vi "Planta de Nivel.vi"() -> ()   [LabVIEW 2020]
uses:
  <vilib>/NI/Modbus Library/API/Wrapper/Create TCP Master.vi
  <vilib>/ErrorRing/Error Ring.xnode
  <vilib>/NI/Modbus Library/API/Master/Modbus Master.lvclass
  <vilib>/NI/Modbus Library/API/Wrapper/API Main.lvlib
panel:
  in  "Vertical Progress Bar":u16(slide) scale=0.0..10.0
  in  "stop":bool
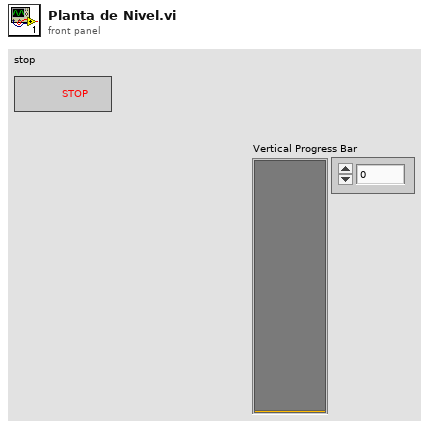
[diagram p1: front panel]
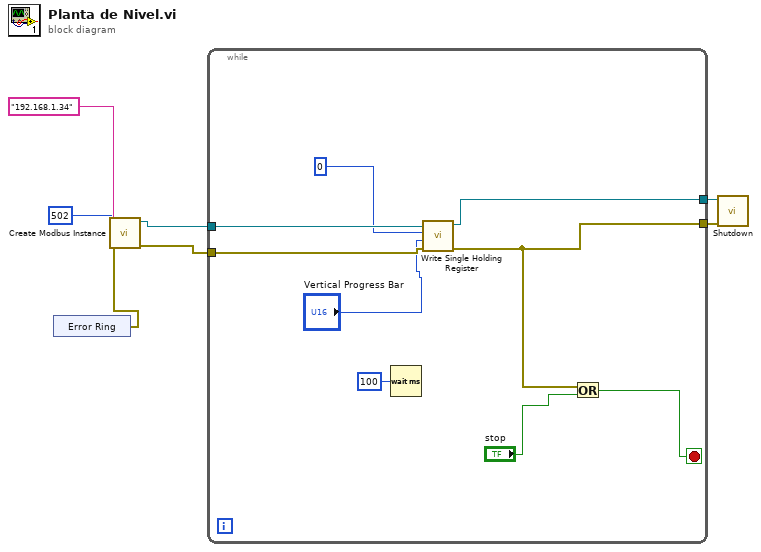
[diagram p0: block diagram]
diagram:
  n1 = xnode "Error Ring"() -> ("error out"=w1:errorcluster)
  n2 = call-poly <vilib>:"Create Modbus Instance.vi"("error in"=w1, "port (502)"=u16 502, "address"="192.168.1.34") -> ("error out"=w4:errorcluster, "TCP master instance"=w5:refnum<class "Modbus Master.lvclass">)  [unwired: 7 in]
  n3 = while {
    tunnel: w5 -> [w15]
    tunnel: w4 -> [w14]
    tunnel: [w13] -> w3
    tunnel: [w10] -> w2
    stop <- w8 stop-if-true
    n4 = Wait (ms)(milliseconds to wait=u32 100) -> ()  [unwired: 1 out]
    n5 = call-dynamic "Write Single Holding Register.vi"("error in"=w14, "register to write"="Vertical Progress Bar", "address"=u16 0, "Modbus master in"=w15) -> ("error out"=w10:errorcluster, "Modbus master out"=w13:refnum<class "Modbus Master.lvclass">)  [unwired: 6 in]
    n6 = Or(x=w10, y="stop") -> (x .or. y?=w8:bool)
  }
  n7 = call-dynamic "Shutdown.vi"("error in"=w2, "Modbus master in"=w3) -> ()  [unwired: 9 in, 1 out]
